vi "P8.vi"() -> ()   [LabVIEW 2018]
panel:
  out "error IO":errorcluster
  out "2D Picture":picture
  out "data":string
  in  "error in (no error)":errorcluster
  in  "UR de la imagen":string
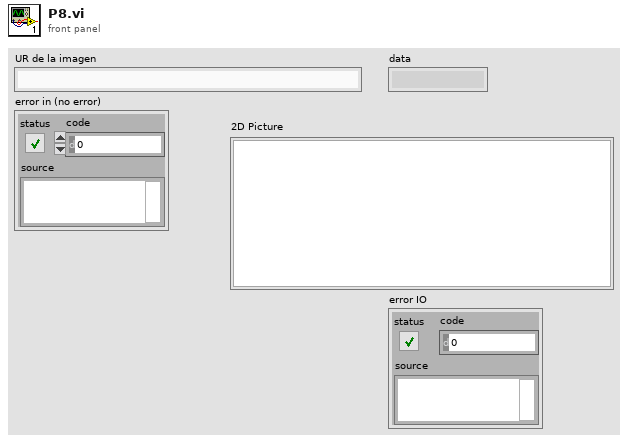
[diagram p1: front panel]
types:
  T1 = enum16{"open", "replace", "create", "open or create", "replace or create", "replace or create with confirmation"}
  T2 = typedef "imagedata.ctl" = cluster{"image type":i32, "image depth":i32, "image":u8[], "mask":u8[], "colors":u32[], "Rectangle":cluster{"left":i16, "top":i16, "right":i16, "bottom":i16}}
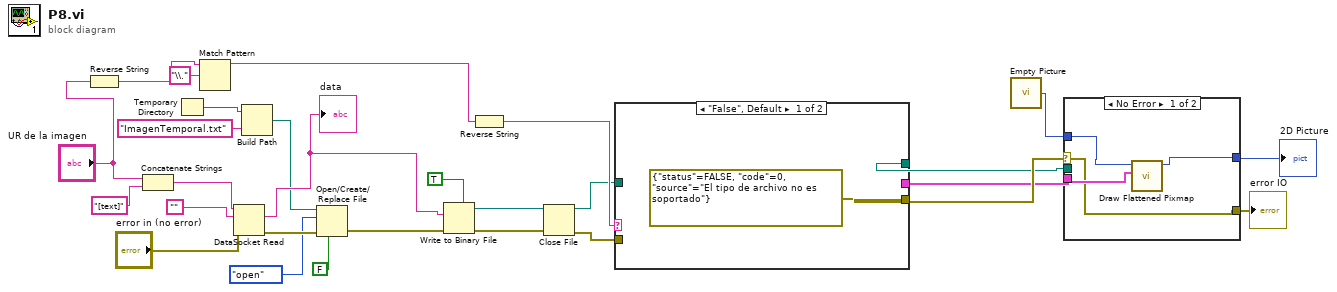
[diagram p0: block diagram]
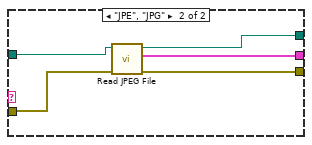
[diagram p3: hidden frame]
diagram:
  n1 = Reverse String(1:"UR de la imagen") -> (0:w16:string)
  n2 = Concatenate Strings("UR de la imagen", "[text]" ("string")) -> (w28:string)
  n3 = Temporary Directory() -> (w14:path)
  n4 = Match Pattern(string=w16, regular expression="\\.") -> (before substring=w10:string)  [unwired: 1 in, 3 out]
  n5 = DataSocket Read(8:"error in (no error)", 10:"", 11:w28) -> (0:w25:errorcluster, 2:w18:string)  [unwired: 2 in, 5 out]
  "data" <- w18
  n6 = Build Path(base path=w14, name or relative path="ImagenTemporal.txt") -> (appended path=w12:path)
  n7 = Open/Create/Replace File(file path (use dialog)=w12, error in=w25, operation (0:open)=T1."open", disable buffering (F)=FALSE) -> (error out=w20:errorcluster)  [unwired: 2 in, 2 out]
  n8 = Write to Binary File(data=w18, error in=w20, 5:TRUE ("prepend array or string size? (T)")) -> (refnum out=w22:refnum<file>, error out=w21:errorcluster)  [unwired: 3 in, 1 out]
  n9 = Reverse String(1:w10) -> (0:w9:string)
  n10 = Close File(refnum=w22, error in=w21) -> (path=w8:path, error out=w7:errorcluster)
  n11 = case shown="\"False\", Default" w9 {
    tunnel: w8 -> [_ w34]
    tunnel: w7 -> [_ w33]
    tunnel: [_ w32] -> w5
    tunnel: [_ w31] -> w4
    tunnel: [errorcluster {"status"=FALSE, "code"=0, "source"="El tipo de archivo no es soportado"} ("error out") w30] -> w6
    frame "False", Default {
    }
    frame "JPE", "JPG" {
      n12 = call <vilib>:"Read JPEG File.vi"("error in (no error)"=w33, "path to JPEG file"=w34) -> ("error out"=w30:errorcluster, "image data"=w32:T2, "path"=w31:path)  [unwired: 7 in]
    }
  }
  n13 = call "Empty Picture"() -> ("empty picture"=w3:picture)
  n14 = case shown="No Error" w6 {
    selector: w6 -> [w35 w40]
    tunnel: w5 -> [w38 _]
    tunnel: w4 -> [_ _]
    tunnel: w3 -> [w37 w39]
    tunnel: [w36 w39] -> w2
    tunnel: [w35 w40] -> w1
    frame No Error {
      n15 = call <vilib>:"Draw Flattened Pixmap.vi"("image data"=w38, "picture"=w37) -> ("new picture"=w36:picture)  [unwired: 7 in]
    }
    frame Error {
    }
  }
  "2D Picture" <- w2
  "error IO" <- w1
